vi "db_data_input_b2g1_MR_gas_meas.vi"() -> ()   [LabVIEW 2011]
uses:
  <vilib>/Platform/TimedLoop/XDataNode/timing_clust.ctl
  <vilib>/Platform/TimedLoop/XDataNode/nitl_modes.ctl
  <vilib>/Platform/TimedLoop/XDataNode/wakeup.ctl
  <vilib>/addons/database/Connection.llb/DB Tools Open Connec (Path).vi
  <vilib>/Platform/TimedLoop/XDataNode/XDataNode.xnode
  <vilib>/addons/database/_DB Variant To Data/Database Variant To Data.xnode
  <vilib>/Platform/TimedLoop/XDataNode/XDNodeRunTimeDep.lvlib
  <vilib>/addons/database/NI_Database_API.lvlib
panel:
  in  "H2 [%]":dbl format="%.2g"
  in  "CO2 [%]":dbl format="%.2g"
  in  "CH4 [%]":dbl format="%.2g"
  in  "pressure [mbar]":dbl format="%.2g"
  in  "temp. [°C]":dbl format="%.2g"
  in  "send data":bool
  in  "volume [l]":dbl format="%.2g"
  in  "sampling timestamp":timestamp format="%<%X\n%x>T"
  in  "Reload":bool
  out "B2G1_MR_gas_meas":string[][](table)
  in  "stop":bool
  # "Write gas measurement data of B2G1_MR to the database"
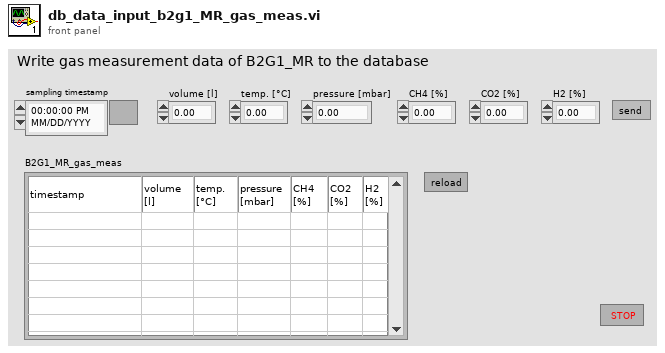
[diagram p1: front panel]
types:
  T1 = typedef "NI_Database_API.lvlib/Conn ObjectReference.ctl" = refnum<k1>
  T2 = typedef "XDNodeRunTimeDep.lvlib/timing_clust.ctl" = cluster{"Expected End [f-1]":u64, "Actual End [f-1]":u64, "Finished Late? [f-1]":bool, "Expected End [i-1]":u64, "Actual End [i-1]":u64, "Finished Late? [i-1]":bool, "Expected Start [i]":u64, "Actual Start [i]":u64, "Expected Start [f]":u64, "Actual Start [f]":u64, "Source Name":string, "Structure Name":string, "Period":i64, "Deadline":i64, "Offset":i64, "Start":i64, "Priority":i32, "Timeout":i32, "Mode":T3, "Wakeup Reason":T4, "Error":errorcluster, "Source Type":string, "Secondary Source Type":string, "Global End Time":u64, "Global Start Time":u64, "Frame Duration":u64, "Iteration Duration":u64, "Assigned CPU":i32, "I/O Scan Engine Mode":u32}
  T3 = typedef "XDNodeRunTimeDep.lvlib/nitl_modes.ctl" = enum32{"No Change", "Process missed periods, maintain original phase", "Discard missed periods, maintain original phase", "Process missed periods, ignore original phase", "Discard missed periods, ignore original phase"}
  T4 = typedef "XDNodeRunTimeDep.lvlib/wakeup.ctl" = enum32{"Normal", "Aborted", "Asynchronous wakeup", "Timing source error", "Timed loop error", "Timeout"}
  T5 = cluster{"sampling timestamp":timestamp, "volume [l]":dbl, "temp. [°C]":dbl, "pressure [mbar]":dbl, "CH4 [%]":dbl, "CO2 [%]":dbl, "H2 [%]":dbl}
  T6 = enum32{"invalid app kind", "Development System", "Run Time System", "Student Edition", "Embedded LabVIEW", "Evaluation", "Custom"}
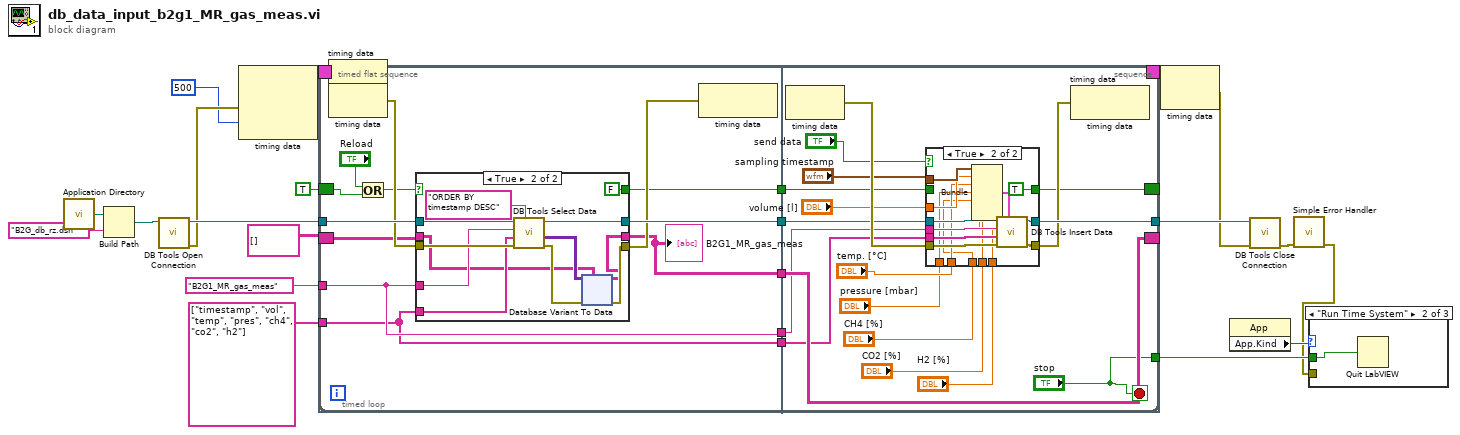
[diagram p0: block diagram]
diagram:
  n1 = call <vilib>:"Application Directory.vi"() -> ("Application Directory"=w3:path)
  n2 = Build Path(base path=w3, name or relative path="B2G_db_rz.dsn" ("Name of ini file 2")) -> (appended path=w1:path)
  n3 = call-poly <vilib>:"DB Tools Open Connection.vi"("connection information"=w1) -> ("error out"=w16:errorcluster, "connection reference"=w18:T1)  [unwired: 7 in]
  n4 = node-c288(w16, i64 500 ("Period")) -> (w10:T2)  [unwired: 1 in]
  n5 = timed-loop {
    timing: w10 -> [_]
    timing-out: [_] -> w9
    tunnel: w18 -> [w27]
    tunnel: [w26] -> w17
    tunnel: "B2G1_MR_gas_meas" ("table") -> [w25]
    tunnel: string[] ["timestamp", "vol", "temp", "pres", "ch4", "co2", "h2"] ("columns") -> [w24]
    shift-right: [w23] -> _
    shift-left: string[][] [] ("data") -> [w22]
    shift-right: [w21] -> _
    shift-left: TRUE -> [w20]
    tunnel: [w19] -> w7
    stop <- "stop" stop-if-true
    n6 = timed-sequence {
      timing: _ -> [_]
      timing-out: _ -> [_]
      tunnel: w27 -> [w41]
      tunnel: [w40] -> w26
      tunnel: w25 -> [w39]
      tunnel: w24 -> [w38]
      tunnel: [w32] -> w23
      tunnel: w22 -> [w31]
      tunnel: [w30] -> w21
      tunnel: w20 -> [w29]
      tunnel: [w28] -> w19
      n7 = timed-flat-sequence {
        tunnel: w41 -> [w53]
        tunnel: [w51] -> w37
        tunnel: [w49] -> w36
        tunnel: [w46] -> w35
        tunnel: w39 -> [w44]
        tunnel: w38 -> [w43]
        tunnel: [w44] -> w34
        tunnel: [w43] -> w33
        tunnel: w31 -> [w45]
        tunnel: w29 -> [w48]
        tunnel: [w136] -> w40
        tunnel: w37 -> [w133]
        tunnel: w36 -> [w125]
        tunnel: w35 -> [w132]
        tunnel: w34 -> [w131]
        tunnel: w33 -> [w130]
        tunnel: [w132] -> w32
        tunnel: [w126] -> w30
        tunnel: ["stop"] -> w28
        frame #0 {
          n8 = node-c288() -> (w52:errorcluster)  [unwired: 1 in]
          n9 = Or(x="Reload", y=w48) -> (x .or. y?=w42:bool)
          n10 = case shown="True" w42 {
            selector: w42 -> [w55 _]
            tunnel: w53 -> [w57 w69]
            tunnel: w52 -> [w56 w68]
            tunnel: [w57 w67] -> w51
            tunnel: [w56 w64] -> w50
            tunnel: [w54 w63] -> w46
            tunnel: [w55 FALSE] -> w49
            tunnel: w45 -> [w54 w58]
            tunnel: w44 -> [_ w61]
            tunnel: w43 -> [_ w60]
            frame False {
            }
            frame True {
              n11 = call <vilib>:"DB Tools Select Data.vi"("condition"="ORDER BY timestamp DESC", "error in (no error)"=w68, "columns"=w60, "table"=w61, "connection reference"=w69) -> ("error out"=w65:errorcluster, "data"=w66:variant[][], "connection reference out"=w67:T1)  [unwired: 1 in]
              n12 = xnode "Database Variant To Data"("database variant"=w66, "error in"=w65, "type"=w58) -> ("data"=w63:string[][], "error out"=w64:errorcluster)
            }
          }
          "B2G1_MR_gas_meas" <- w46
          n13 = node-c288(w50) -> ()  [unwired: 1 out]
        }
        frame #1 {
          n14 = node-c288() -> (w135:errorcluster)  [unwired: 1 in]
          n15 = case shown="True" "send data" {
            tunnel: [w138 w154] -> w136
            tunnel: w135 -> [w137 w153]
            tunnel: [w137 w152] -> w134
            tunnel: w133 -> [w138 w151]
            tunnel: w131 -> [_ w150]
            tunnel: w130 -> [_ w149]
            tunnel: "sampling timestamp" -> [_ w148]
            tunnel: "volume [l]" -> [_ w147]
            tunnel: [w139 TRUE] -> w126
            tunnel: w125 -> [w139 _]
            tunnel: "temp. [°C]" -> [_ w144]
            tunnel: "pressure [mbar]" -> [_ w143]
            tunnel: "CH4 [%]" -> [_ w142]
            tunnel: "CO2 [%]" -> [_ w141]
            tunnel: "H2 [%]" -> [_ w140]
            frame False {
            }
            frame True {
              n16 = Bundle("sampling timestamp"=w148, "volume [l]"=w147, "temp. [°C]"=w144, "pressure [mbar]"=w143, "CH4 [%]"=w142, "CO2 [%]"=w141, "H2 [%]"=w140) -> (w146:T5)  [unwired: 1 in]
              n17 = call <vilib>:"DB Tools Insert Data.vi"("data"=w146, "error in (no error)"=w153, "columns"=w149, "table"=w150, "connection reference"=w151) -> ("error out"=w152:errorcluster, "connection reference out"=w154:T1)  [unwired: 5 in]
            }
          }
          n18 = node-c288(w134) -> ()  [unwired: 1 out]
        }
      }
    }
    n19 = node-c288() -> ()  [unwired: 1 in, 1 out]
    n20 = node-c288() -> ()  [unwired: 1 in, 1 out]
  }
  n21 = node-c288(w9) -> (w15:errorcluster)
  n22 = property class="App"() -> ("App.Kind"=w5:T6)  [unwired: 2 in, 2 out]
  n23 = call <vilib>:"DB Tools Close Connection.vi"("error in (no error)"=w15, "connection reference"=w17) -> ("error out"=w6:errorcluster)  [unwired: 5 in]
  n24 = call <vilib>:"Simple Error Handler.vi"("error in (no error)"=w6) -> ("error out"=w4:errorcluster)  [unwired: 4 in, 4 out]
  n25 = case shown="\"Run Time System\"" w5 {
    tunnel: w7 -> [_ w162 _]
    tunnel: w4 -> [_ _ _]
    frame "invalid app kind", Default {
    }
    frame "Run Time System" {
      n26 = Quit LabVIEW(quit? (T)=w162) -> ()
    }
    frame "Development System" {
    }
  }
